vi "Shutdown.vi"(8 "error in (no error)":errorcluster, 11 "MB CR in":refnum<class "Modbus Master CR API.lvclass">) -> (0 "error out":errorcluster)   [LabVIEW 2021, in "Modbus Master CR API.lvclass"]
doc: "Closes and destroys a Modbus slave instance."
uses:
  Modbus Master CR API.lvclass
  Modbus Master CR API.lvclass/Modbus Master CR API.ctl
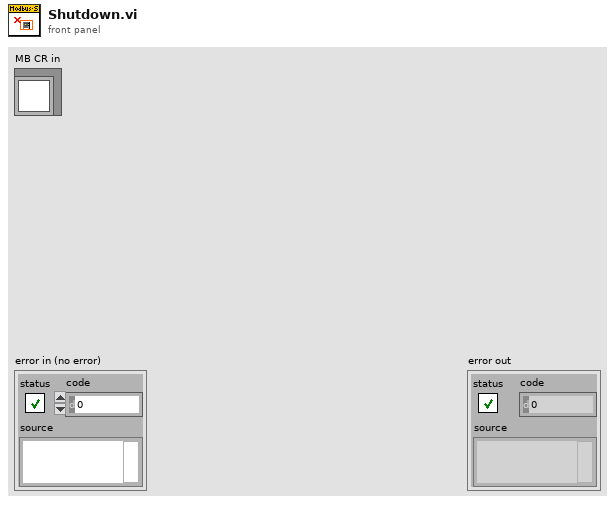
[diagram p1: front panel]
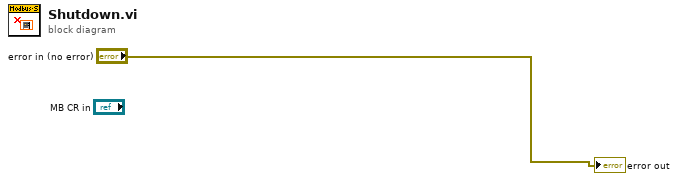
[diagram p0: block diagram]
diagram:
  "error out" <- "error in (no error)"
